vi "Main GUI.vi"(8 "error in (no error)":errorcluster, 11 "Simple Build GUI in":refnum<class "Simple Build GUI.lvclass">) -> (0 "error out":errorcluster, 3 "Simple Build GUI out":refnum<class "Simple Build GUI.lvclass">)   [LabVIEW 2020, in "Builder Tools.lvlib" / "Simple Build GUI.lvclass"]
uses:
  Simple Build GUI.lvclass
  Builder Core/Version Type.ctl
  Simple Build GUI.lvclass/Simple Build GUI.ctl
  Builder Core/Builder Core.lvlib
  Builder/Builder.lvclass
panel:
  out "Message":string
  out "Log":string
  out "Progress":i32(slide) scale=0.0..100.0
  in  "Build":bool
  in  "Pre-Release (None)":string
  out "Next Version":string
  in  "Version Type":T1=enum."Fix"
  out "Current Version":string
  in  "Builds":T2(array[cluster])
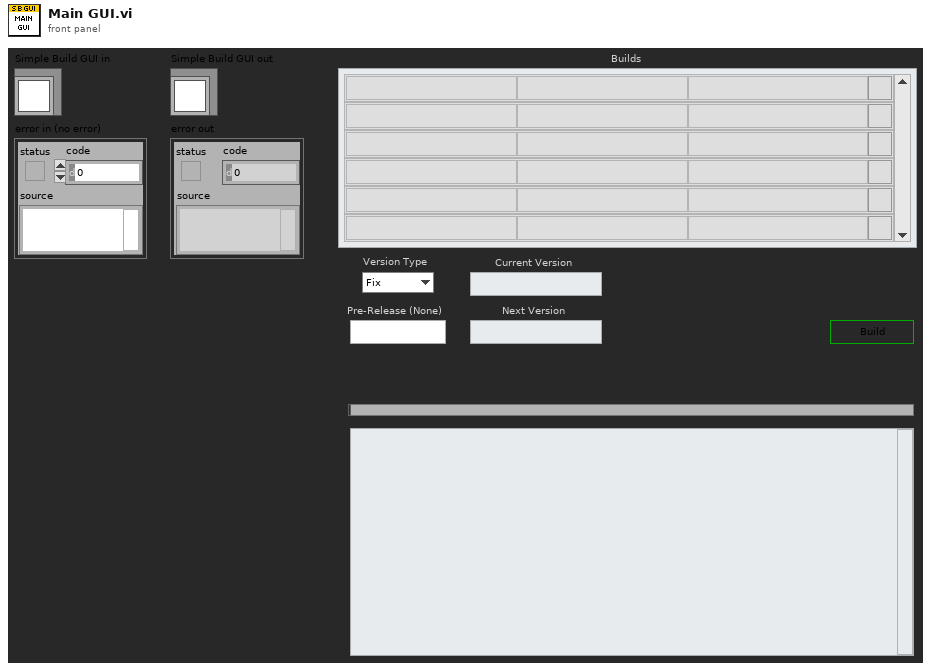
[diagram p1: front panel]
types:
  T1 = typedef "Builder Core.lvlib/Version Type.ctl" = enum16{"None", "Fix", "Minor", "Major"}
  T2 = cluster{"Project":string, "Target":string, "Build Spec":string, "Build":bool}[]
  T3 = enum8{"Enabled", "Disabled", "Disabled and Grayed Out"}
  T4 = typedef "LVRectTypeDef.ctl" = cluster{"Left":i16, "Top":i16, "Right":i16, "Bottom":i16}
  T5 = typedef "Builder Core.lvlib/Version.ctl" = cluster{"Major":u16, "Minor":u16, "Fix":u16, "Build":u16}
  T6 = typedef "Builder Tools.lvlib/Simple Build GUI.lvclass/Build Info.ctl" = cluster{"Project":string, "Target":string, "Build Spec":string, bool}
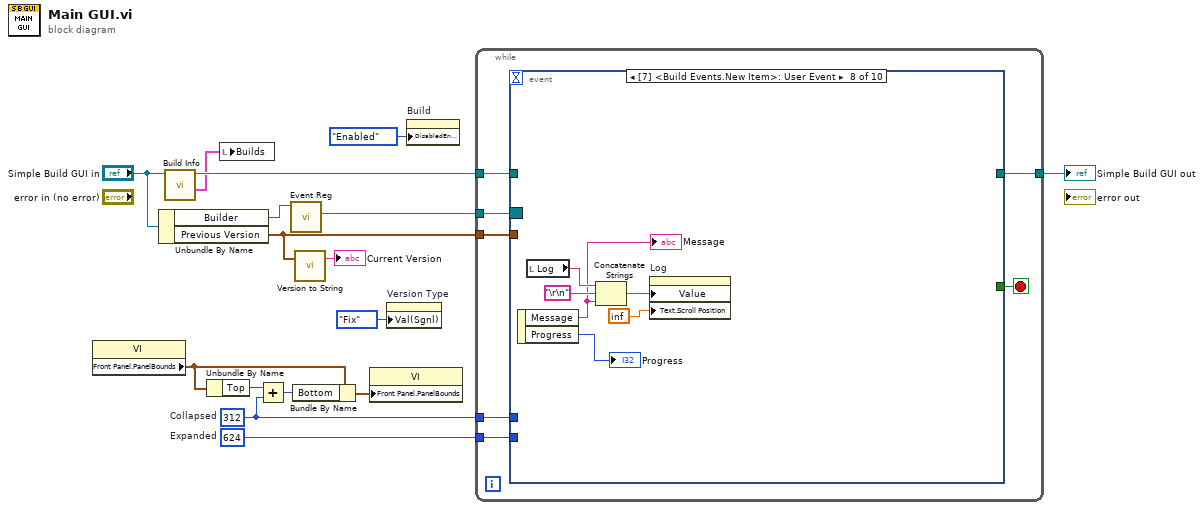
[diagram p0: block diagram]
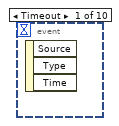
[diagram p2: hidden frame]
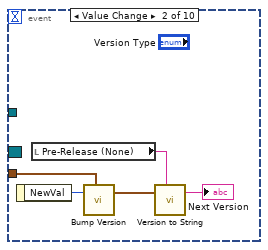
[diagram p3: hidden frame]
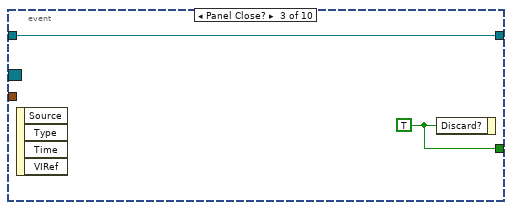
[diagram p4: hidden frame]
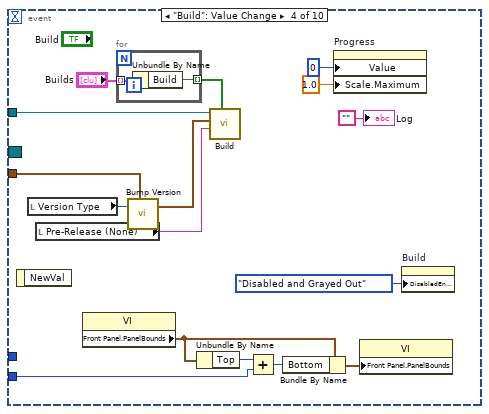
[diagram p5: hidden frame]
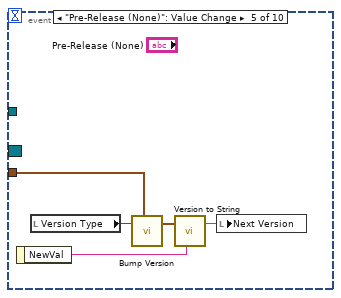
[diagram p6: hidden frame]
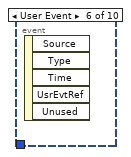
[diagram p7: hidden frame]
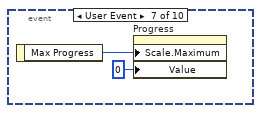
[diagram p8: hidden frame]
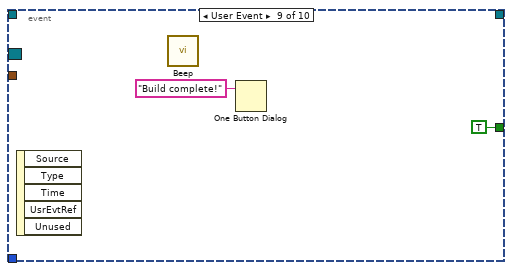
[diagram p9: hidden frame]
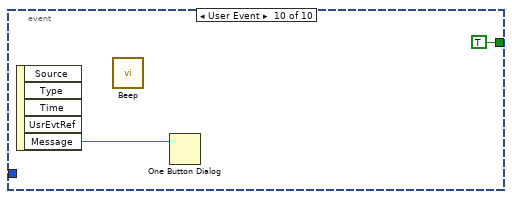
[diagram p10: hidden frame]
diagram:
  w6 = i16 624  # Expanded
  w7 = i16 312  # Collapsed
  n1 = property class="VI"() -> ("Front Panel.PanelBounds"=w10:T4)  [unwired: 2 in, 2 out]
  n2 = Unbundle By Name("Simple Build GUI in") -> ("Builder"=w4:refnum<class "Builder.lvclass">, "Previous Version"=w13:T5)
  n3 = call "Build Info.vi"("Simple Build GUI in"="Simple Build GUI in") -> ("Builds"=w1:T6[], "Simple Build GUI out"=w2:refnum<class "Simple Build GUI.lvclass">)  [unwired: 7 in, 2 out]
  n4 = Unbundle By Name(w10) -> ("Top"=w11:i16)
  n5 = local write "Builds"(w1) -> ()
  n6 = Add(x=w11, y=w7) -> (x+y=w9:i16)
  n7 = call "Event Reg.vi"("Builder in"=w4) -> ("Event Reg"=w3:refnum<event-registration>)  [unwired: 9 in, 1 out]
  n8 = Bundle By Name(cluster=w10, "Bottom"=w9) -> (w8:T4)
  n9 = call "Version to String.vi"("Version"=w13) -> ("Version String"=→"Current Version":string)  [unwired: 6 in]
  n10 = property class="VI"("Front Panel.PanelBounds"=w8) -> ()  [unwired: 2 in, 2 out]
  n11 = property on="Version Type" class="Enum (strict)"("Val(Sgnl)"=Version_Type."Fix" ("Value (Signaling)")) -> ()  [unwired: 2 in, 2 out]
  n12 = property on="Build" class="Bool"("DisabledEnum"=T3."Enabled" ("Disabled")) -> ()  [unwired: 2 in, 2 out]
  n13 = while {
    tunnel: w2 -> [w23]
    tunnel: w13 -> [w22]
    tunnel: [w20] -> w12
    tunnel: w7 -> [w19]
    tunnel: w6 -> [w18]
    tunnel: w3 -> [w17]
    stop <- w21 stop-if-true
    n14 = event shown="[7] <Build Events.New Item>: User Event" {
      selector: w17 -> [_ _ _ _ _ _ _ _ _ _]
      dyn-events: _ -> [_ _ _ _ _ _ _ _ _ _]
      timeout: _ -> [_ _ _ _ _ _ _ _ _ _]
      tunnel: w23 -> [_ _ w29 w41 _ _ _ _ _ _]
      tunnel: w22 -> [_ w28 _ w43 w52 _ _ _ _ _]
      tunnel: [_ _ w30 _ _ _ _ _ TRUE ("Discard?") TRUE ("Discard?")] -> w21
      tunnel: [_ _ w29 _ _ _ _ _ _ _] -> w20
      tunnel: w19 -> [_ _ _ _ _ _ _ _ _ _]
      tunnel: w18 -> [_ _ _ w34 _ _ _ _ _ _]
      event Timeout {
        n15 = event-data() -> ()  [unwired: 1 in, 3 out]
      }
      event Value Change {
        n16 = event-data() -> ("NewVal"=w27:T1)  [unwired: 1 in]
        n17 = local read "Pre-Release (None)"() -> (w24:string)
        n18 = call "Bump Version.vi"("Version Type"=w27, "Previous Version"=w28) -> ("Next Version"=w26:T5)  [unwired: 5 in]
        n19 = call "Version to String.vi"("Version"=w26, "Pre-Release (None)"=w24) -> ("Version String"=→"Next Version":string)  [unwired: 5 in]
      }
      event Panel Close? {
        w30 = TRUE ("Discard?")
        n20 = event-data() -> ()  [unwired: 1 in, 4 out]
        n21 = event-data("Discard?"=w30) -> ()  [unwired: 1 in, 1 out]
      }
      event "Build": Value Change {
        n22 = event-data() -> ()  [unwired: 1 in, 1 out]
        n23 = local read "Version Type"() -> (w42:T1)
        n24 = local read "Pre-Release (None)"() -> (w39:string)
        n25 = property class="VI"() -> ("Front Panel.PanelBounds"=w36:T4)  [unwired: 2 in, 2 out]
        n26 = for {
          tunnel: "Builds" -> [w48] mode=indexing
          tunnel: [w47] -> w32 mode=indexing
          n27 = Unbundle By Name(w48) -> ("Build"=w47:bool)
        }
        n28 = call "Bump Version.vi"("Version Type"=w42, "Previous Version"=w43) -> ("Next Version"=w40:T5)  [unwired: 5 in]
        n29 = Unbundle By Name(w36) -> ("Top"=w35:i16)
        n30 = call "Build.vi"("Build"=w32, "Pre-Release"=w39, "Version"=w40, "Simple Build GUI in"=w41) -> ()  [unwired: 6 in, 2 out]
        n31 = Add(x=w35, y=w34) -> (x+y=w37:i16)
        n32 = Bundle By Name(cluster=w36, "Bottom"=w37) -> (w38:T4)
        n33 = property on="Progress" class="Slide (strict)"("Value"=0 ("Progress"), "Scale.Maximum"=1.0 ("Scale.Range:Maximum")) -> ()  [unwired: 2 in, 2 out]
        n34 = property class="VI"("Front Panel.PanelBounds"=w38) -> ()  [unwired: 2 in, 2 out]
        n35 = property on="Build" class="Bool"("DisabledEnum"=T3."Disabled and Grayed Out" ("Disabled")) -> ()  [unwired: 2 in, 2 out]
        "Log" <- "" ("Log")
      }
      event "Pre-Release (None)": Value Change {
        n36 = event-data() -> ("NewVal"=w50:string)  [unwired: 1 in]
        n37 = local read "Version Type"() -> (w53:T1)
        n38 = call "Bump Version.vi"("Version Type"=w53, "Previous Version"=w52) -> ("Next Version"=w51:T5)  [unwired: 5 in]
        n39 = call "Version to String.vi"("Version"=w51, "Pre-Release (None)"=w50) -> ("Version String"=w49:string)  [unwired: 5 in]
        n40 = local write "Next Version"(w49) -> ()
      }
      event User Event {
        n41 = event-data() -> ()  [unwired: 1 in, 5 out]
      }
      event User Event {
        n42 = event-data() -> ("Max Progress"=w55:i32)  [unwired: 1 in]
        n43 = property on="Progress" class="Slide (strict)"("Scale.Maximum"=w55, "Value"=0 ("Progress")) -> ()  [unwired: 2 in, 2 out]
      }
      event User Event {
        n44 = event-data() -> ("Message"=w56:string, "Progress"=→"Progress":i32)  [unwired: 1 in]
        "Message" <- w56
        n45 = local read "Log"() -> (w60:string)
        n46 = Concatenate Strings(w60, "\r\n", w56) -> (w58:string)
        n47 = property on="Log" class="Str"("Value"=w58, "Text.Scroll Position"=inf) -> ()  [unwired: 2 in, 2 out]
      }
      event User Event {
        n48 = event-data() -> ()  [unwired: 1 in, 5 out]
        n49 = call <vilib>:"Beep.vi"() -> ()  [unwired: 12 in]
        n50 = One Button Dialog(message="Build complete!") -> ()  [unwired: 1 in, 1 out]
      }
      event User Event {
        n51 = event-data() -> ("Message"=w65:string)  [unwired: 1 in, 4 out]
        n52 = call <vilib>:"Beep.vi"() -> ()  [unwired: 12 in]
        n53 = One Button Dialog(message=w65) -> ()  [unwired: 1 in, 1 out]
      }
    }
  }
  "Simple Build GUI out" <- w12
